vi "Write Wfm Data.vi"(8 "error in (no error)":errorcluster, 11 "Async State Vars in":T1) -> (0 "error out":errorcluster, 3 "Async State Vars out":T1, 4 "Wfm timed out?":bool)   [LabVIEW 2015, in "Waveform-Processing-Custom-Device Engine.lvlib"]
uses:
  Waveform-Processing-Custom-Device Engine.lvlib
  Types/AsyncStateVariables.ctl
  <vilib>/NI Veristand/Custom Device Waveform API/Single Waveform Read (DBL)/Single Waveform Read (DBL).lvclass
  <vilib>/NI Veristand/Custom Device Waveform API/Single Waveform Write (DBL)/Single Waveform Write (DBL).lvclass
  <vilib>/NI Veristand/Custom Device API/Waveform Data Reference.ctl
  <vilib>/ni/NIVS Inline Async API/_Data Access Engine/Data Access Engine/Types/Write.DVR.ctl
  <vilib>/ni/NIVS Inline Async API/_Data Access Engine/Access Type Classes/Write/Write.lvclass
  <vilib>/ni/NIVS Inline Async API/_Data Access Engine/Data Access Engine/Types/Read.DVR.ctl
  <vilib>/ni/NIVS Inline Async API/_Data Access Engine/Access Type Classes/Read/Read.lvclass
  <vilib>/NI Veristand/Custom Device Waveform API/Waveform Session.lvclass/Waveform Session.ctl
  <vilib>/NI Veristand/Custom Device Waveform API/Single Waveform Write (DBL)/Single Waveform Write (DBL).lvclass/Single Waveform Write (DBL).ctl
  <vilib>/NI Veristand/Custom Device Waveform API/Internal Comm Classes/WPL Comm/WPL Comm (1D DBL)/WPL Comm (1D DBL).lvclass/WPL Comm (1D DBL).ctl
  <vilib>/NI Veristand/Custom Device Waveform API/Internal Comm Classes/WPL Comm/WPL Comm.lvclass/WPL Comm.ctl
  <vilib>/NI Veristand/Custom Device Waveform API/Single Waveform Write (DBL)/NI VeriStand - Write Single Waveform (DBL).vi
  <vilib>/NI Veristand/Custom Device Waveform API/Internal Comm Classes/WPL Comm/WPL Comm (1D DBL)/Comm_write 1d dbl.vi
  <vilib>/NI Veristand/Custom Device Waveform API/Read Sample offset DVR.vi
  <vilib>/NI Veristand/Custom Device Waveform API/Check Opened.vi
  <vilib>/NI Veristand/Custom Device Waveform API/Internal Comm Classes/WPL Comm/Direct Send WPL Command.vi
  <vilib>/NI Veristand/Custom Device Waveform API/Internal Comm Classes/WPL Comm/Convert Q Error to Shutdown Error.vi
  <vilib>/Utility/error.llb/Error Cluster From Error Code.vi
  <vilib>/NI Veristand/Custom Device Waveform API/NI_VS Custom Device Waveform API.lvlib
  <vilib>/NI VeriStand/Custom Device API/Custom Device API.lvlib
  <vilib>/ni/NIVS Inline Async API/_Data Access Engine/Data Access Engine/Data Access Engine.lvclass
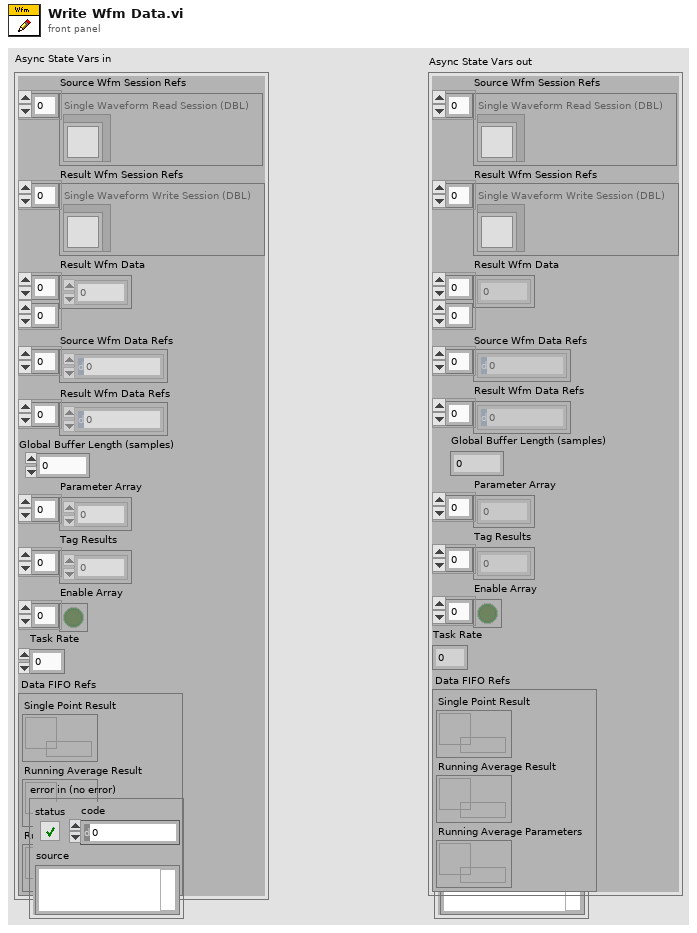
[diagram p1: front panel]
types:
  T1 = typedef "Waveform-Processing-Custom-Device Engine.lvlib/AsyncStateVariables.ctl" = cluster{"Source Wfm Session Refs":refnum<class "Single Waveform Read (DBL).lvclass">[], "Result Wfm Session Refs":refnum<class "Single Waveform Write (DBL).lvclass">[], "Result Wfm Data":dbl[][], "Source Wfm Data Refs":T2[], "Result Wfm Data Refs":T2[], "Global Buffer Length (samples)":dbl, "Parameter Array":dbl[], "Tag Results":dbl[], "Enable Array":bool[], "Task Rate":dbl, "Data FIFO Refs":cluster{"Single Point Result":T3, "Running Average Result":T3, "Running Average Parameters":T4}}
  T2 = typedef "Custom Device API.lvlib/Waveform Data Reference.ctl" = i32
  T3 = typedef "Data Access Engine.lvlib/Data Access Engine.lvclass/Write.DVR.ctl" = refnum<data-value>
  T4 = typedef "Data Access Engine.lvlib/Data Access Engine.lvclass/Read.DVR.ctl" = refnum<data-value>
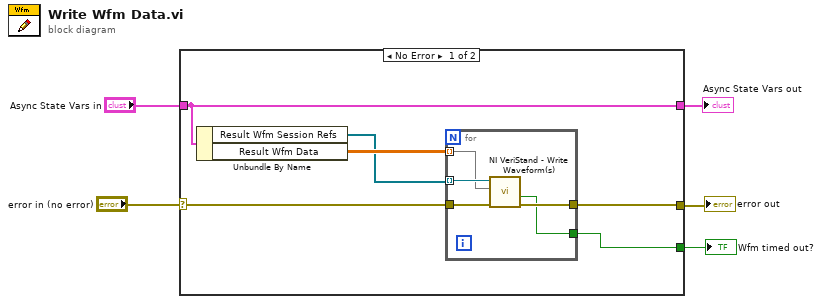
[diagram p0: block diagram]
diagram:
  n1 = case shown="No Error" "error in (no error)" {
    selector: "error in (no error)" -> [w10 w17]
    tunnel: [w11 w17] -> w5
    tunnel: "Async State Vars in" -> [w9 w18]
    tunnel: [w9 w18] -> w2
    tunnel: [w8 _] -> w1
    frame No Error {
      n2 = Unbundle By Name(w9) -> ("Result Wfm Session Refs"=w6:refnum<class "Single Waveform Write (DBL).lvclass">[], "Result Wfm Data"=w7:dbl[][])
      n3 = for {
        tunnel: w10 -> [w16]
        tunnel: [w15] -> w11
        tunnel: [w14] -> w8
        tunnel: w6 -> [w13] mode=indexing
        tunnel: w7 -> [w12] mode=indexing
        n4 = call-poly <vilib>:"NI VeriStand - Write Waveform(s).vi"("error in (no error)"=w16, "Data"=w12, "Single Waveform Write Session (DBL) in"=w13) -> ("error out"=w15:errorcluster, "timed out?"=w14:bool)  [unwired: 6 in, 1 out]
      }
    }
    frame Error {
    }
  }
  "error out" <- w5
  "Wfm timed out?" <- w1
  "Async State Vars out" <- w2
